vi "toml_api_file_write.vi"(8 "error in (no error)":errorcluster, 9 "text":string, 10 "operation (replace or create)":T1(ring)=enum."replace or create", 11 "resolved path":path) -> (0 "error out":errorcluster)   [LabVIEW 2017]
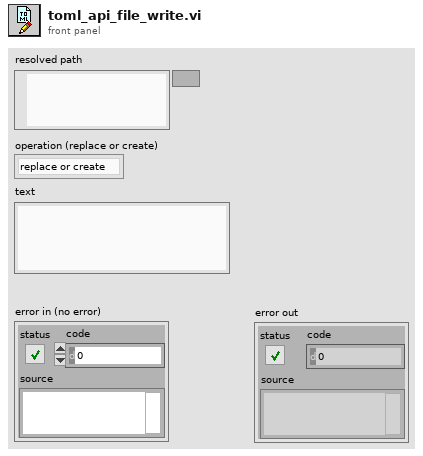
[diagram p1: front panel]
types:
  T1 = enum16{"open", "replace", "create", "open or create", "replace or create", "replace or create with confirmation"}
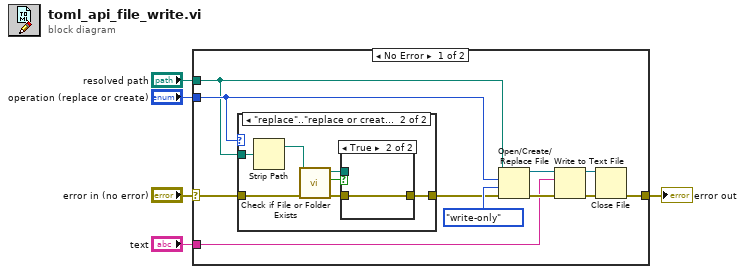
[diagram p0: block diagram]
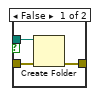
[diagram p3: hidden frame]
diagram:
  n1 = case shown="No Error" "error in (no error)" {
    selector: "error in (no error)" -> [w9 w29]
    tunnel: "resolved path" -> [w7 _]
    tunnel: [w16 w29] -> w3
    tunnel: "operation (replace or create)" -> [w8 _]
    tunnel: "text" -> [w10 _]
    frame No Error {
      n2 = case shown="\"replace\"..\"replace or create with confirmation\"" w8 {
        tunnel: w9 -> [w17 w24]
        tunnel: w7 -> [_ w22]
        tunnel: [w17 w20] -> w6
        frame "open" {
          # "don't create directory"
        }
        frame "replace".."replace or create with confirmation" {
          n3 = Strip Path(path=w22) -> (stripped path=w23:path)  [unwired: 1 out]
          n4 = call <vilib>:"Check if File or Folder Exists.vi"("error in (no error)"=w24, "path"=w23) -> ("error out"=w21:errorcluster, "file or folder exists?"=w18:bool, "dup path"=w19:path)  [unwired: 7 in]
          n5 = case shown="True" w18 {
            tunnel: w21 -> [w27 w28]
            tunnel: [w26 w28] -> w20
            tunnel: w19 -> [w25 _]
            frame False {
              n6 = Create Folder(path (use dialog)=w25, error in=w27) -> (error out=w26:errorcluster)  [unwired: 1 in, 2 out]
            }
            frame True {
            }
          }
        }
      }
      n7 = Open/Create/Replace File(file path (use dialog)=w7, error in=w6, operation (0:open)=w8, access (0:read/write)=enum16{"read/write", "read-only", "write-only"}."write-only") -> (refnum out=w14:refnum<file>, error out=w13:errorcluster)  [unwired: 2 in, 1 out]
      n8 = Write to Text File(file (use dialog)=w14, text=w10, error in=w13) -> (refnum out=w11:refnum<file>, error out=w12:errorcluster)  [unwired: 1 in, 1 out]
      n9 = Close File(refnum=w11, error in=w12) -> (error out=w16:errorcluster)  [unwired: 1 out]
    }
    frame Error {
    }
  }
  "error out" <- w3
